vi "WSVCAP SHL Host TL Status Manager.vi"(11 "error in":errorcluster, 14 "FPGA":T1) -> (4 "System Out":T2={"Settings"={"I2C Slave Address"=144, "I2C Clock Rate (Hz)"=20.0, "SPI Clock Rate (Hz)"=50000.0, "RFFE Slave Address"=255, "RFFE Clock Rate (Hz)"=20.0, "Simulate FPGA"=TRUE, "C1 Cap DAC Default"=165, "C2 Cap DAC Default"=165, "C3 Cap DAC Default"=134, "C4 Cap DAC Default"=150}, "FPGA Resource"="", "Online"=FALSE, "I2C Wait Ticks"=0, "SPI Wait Ticks"=0, "RFFE Wait Ticks"=0, "FPGA VI Reference (FPGA Mode)"=refnum, "FPGA VI Reference (Sim Mode)"=refnum} {"Settings"."C4 Cap DAC Default" format="0x%02x"; "Settings"."C3 Cap DAC Default" format="0x%02x"; "Settings"."C2 Cap DAC Default" format="0x%02x"; "Settings"."C1 Cap DAC Default" format="0x%02x"; "Settings"."RFFE Clock Rate (Hz)" format="%.0f Hz"; "Settings"."RFFE Slave Address" format="0x%02x"; "Settings"."I2C Clock Rate (Hz)" format="%.0f Hz"; "Settings"."SPI Clock Rate (Hz)" format="%.0f Hz"; "Settings"."I2C Slave Address" format="0x%02x"}, 15 "error out":errorcluster)   [LabVIEW 2017]
uses:
  Type Defs/WSVCAP SHL Core System Cluster.ctl
  Type Defs/WSVCAP SHL I2C Settings Cluster.ctl
  Type Defs/WSVCAP SHL FPGA Ref.ctl
  Type Defs/WSVCAP SHL FPGA Enum.ctl
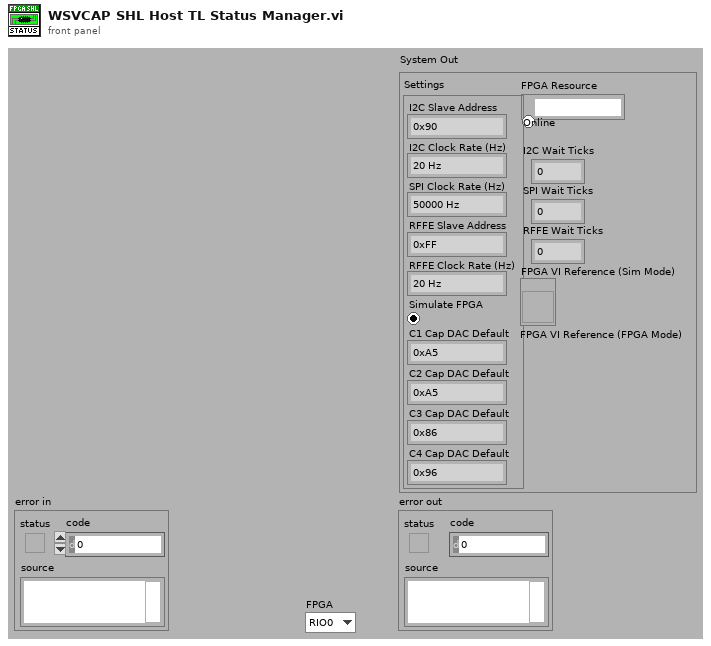
[diagram p1: front panel]
types:
  T1 = typedef "WSVCAP SHL FPGA Enum.ctl" = enum16{"RIO0", "RIO1"}
  T2 = typedef "WSVCAP SHL Core System Cluster.ctl" = cluster{"Settings":T3, "FPGA Resource":tag, "Online":bool, "I2C Wait Ticks":u32, "SPI Wait Ticks":u32, "RFFE Wait Ticks":u32, "FPGA VI Reference (FPGA Mode)":T4, "FPGA VI Reference (Sim Mode)":refnum<vi>}
  T3 = typedef "WSVCAP SHL I2C Settings Cluster.ctl" = cluster{"I2C Slave Address":u8, "I2C Clock Rate (Hz)":dbl, "SPI Clock Rate (Hz)":dbl, "RFFE Slave Address":u8, "RFFE Clock Rate (Hz)":dbl, "Simulate FPGA":bool, "C1 Cap DAC Default":u8, "C2 Cap DAC Default":u8, "C3 Cap DAC Default":u8, "C4 Cap DAC Default":u8}
  T4 = typedef "WSVCAP SHL FPGA Ref.ctl" = refnum<k20>
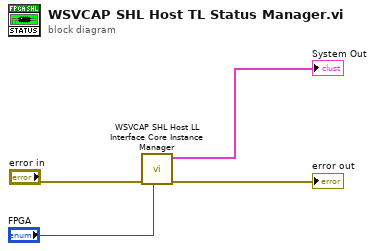
[diagram p0: block diagram]
diagram:
  n1 = call "WSVCAP SHL Host LL Interface Core Instance Manager.vi"("FPGA"="FPGA", "error in (no error)"="error in") -> ("error out"=→"error out":errorcluster, "FGPA Interface Out"=→"System Out":T2)  [unwired: 8 in]
